vi "Close Connection.vi"(8 "error in (no error)":errorcluster, 11 "RemoteControl.STM in":refnum<class "RemoteControl.STM.lvclass">) -> (0 "error out":errorcluster, 3 "RemoteControl.STM out":refnum<class "RemoteControl.STM.lvclass">)   [LabVIEW 2019, in "RemoteControl.STM.lvclass"]
uses:
  RemoteControl.STM.lvclass
  <vilib>/NI/STM/TCP/TCP Connection Info.ctl
  <vilib>/NI/STM/SubVIs/MetaDataElement.ctl
  RemoteControl.STM.lvclass/RemoteControl.STM.ctl
  <vilib>/NI/STM/TCP/Get Connection Reference (TCP).vi
  <vilib>/NI/STM/NI STM.lvlib
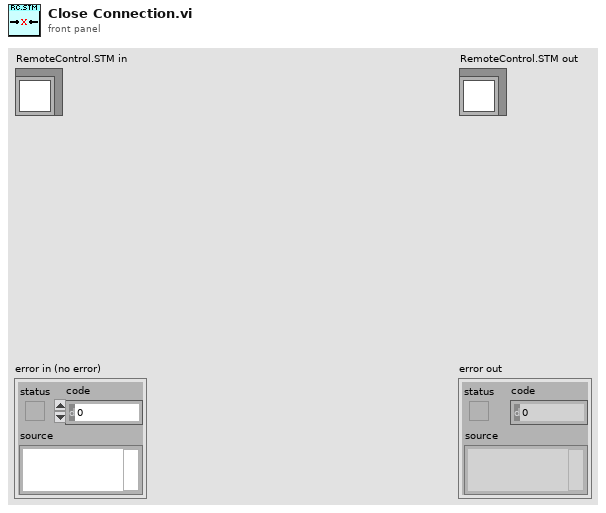
[diagram p1: front panel]
types:
  T1 = typedef "NI STM.lvlib/TCP Connection Info.ctl" = cluster{"connection ID":refnum<k5>, "meta data":T2[]}
  T2 = typedef "NI STM.lvlib/MetaDataElement.ctl" = string
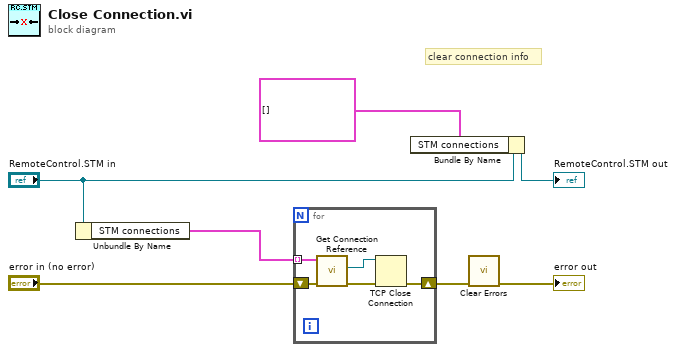
[diagram p0: block diagram]
diagram:
  # "clear connection info"
  n1 = Unbundle By Name("RemoteControl.STM in") -> ("STM connections"=w1:T1[])
  n2 = for {
    tunnel: [w8] -> _ mode=indexing
    shift-right: [w9] -> w4
    shift-left: "error in (no error)" -> [w10]
    tunnel: w1 -> [w8] mode=indexing
    n3 = call-poly <vilib>:"Get Connection Reference.vi"("error in"=w10, "connection info in"=w8) -> ("error out"=w11:errorcluster, "connection ID out"=w12:refnum<k5>)  [unwired: 7 in, 1 out]
    n4 = TCP Close Connection(connection ID=w12, error in (no error)=w11) -> (error out=w9:errorcluster)  [unwired: 1 in, 1 out]
  }
  n5 = Bundle By Name(cluster="RemoteControl.STM in", "STM connections"=T1[] [] ("STM connection info")) -> (→"RemoteControl.STM out":refnum<class "RemoteControl.STM.lvclass">)
  n6 = call <vilib>:"Clear Errors.vi"("error in (no error)"=w4) -> ("error out"=→"error out":errorcluster)  [unwired: 5 in, 1 out]
